vi "Read Sweep configuration.vi"(8 "error in (no error)":errorcluster, 11 "Sweeper  in":refnum<class "Sweeper.lvclass">) -> (0 "error out":errorcluster, 2 "Configuration":T1 {"Sweep  rate" format="%#_6p"; "End sweep" format="%#_6p"; "Start sweep" format="%#_6p"}, 3 "Sweeper  out":refnum<class "Sweeper.lvclass">)   [LabVIEW 2016, in "Sweeper.lvclass"]
uses:
  Sweeper.lvclass
  C:/github/Measure_core/Measure Object/Da Base.lvclass
  NHMFL_Core/Libraries/Instruments/Instrument Driver/Sweeper Driver/Sweep Configuration.ctl
  Measure_core/Da Base/Da Base.lvclass/Da Base.ctl
  Measure_core/Da Base/Read Configuration.vi
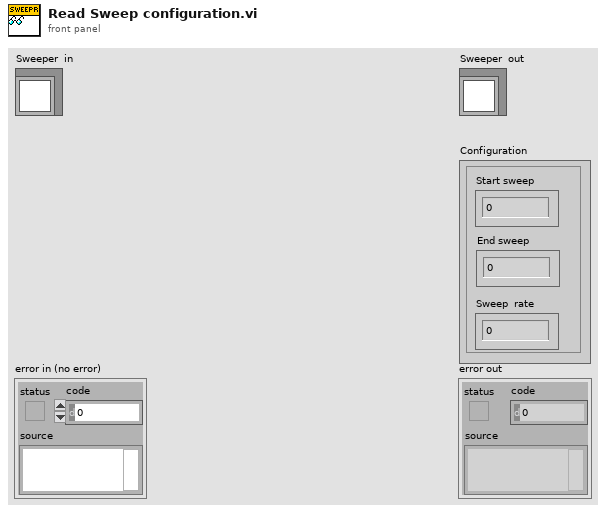
[diagram p1: front panel]
types:
  T1 = typedef "Sweep Configuration.ctl" = cluster{"Start sweep":dbl, "End sweep":dbl, "Sweep  rate":dbl}
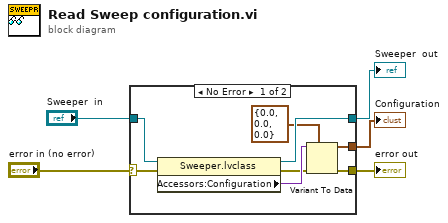
[diagram p0: block diagram]
diagram:
  n1 = case shown="No Error" "error in (no error)" {
    selector: "error in (no error)" -> [w7 w14]
    tunnel: [w11 w14] -> w4
    tunnel: [w12 w15] -> w2
    tunnel: "Sweeper  in" -> [w13 w15]
    tunnel: [w8 _] -> w1
    frame No Error {
      n2 = property class="Sweeper.lvclass"(reference=w13, error in=w7) -> (reference out=w12:refnum<class "Sweeper.lvclass">, error out=w6:errorcluster, "Accessors:Configuration"=w9:variant)
      n3 = Variant To Data(error in=w6, type=T1 {"Start sweep"=0.0, "End sweep"=0.0, "Sweep  rate"=0.0} ("Configuration"), Variant=w9) -> (data=w8:T1, error out=w11:errorcluster)
    }
    frame Error {
    }
  }
  "error out" <- w4
  "Sweeper  out" <- w2
  "Configuration" <- w1
